vi "MSScript_Transform_Boolean.vi"(11 "Check_Str":string) -> (2 "Value Error?":bool, 3 "Value Output":bool)   [LabVIEW 2018, in "MSScript.lvclass"]
uses:
  MSScript.lvclass
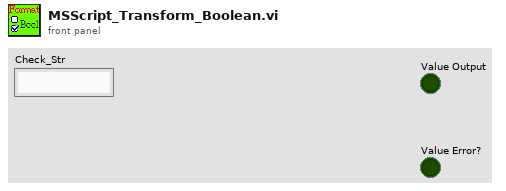
[diagram p1: front panel]
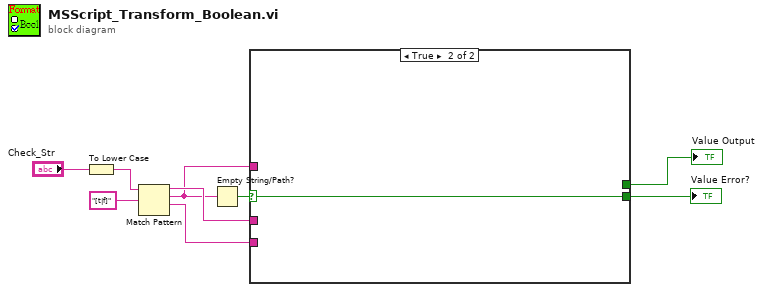
[diagram p0: block diagram]
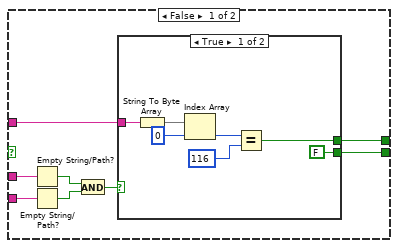
[diagram p2: hidden frame]
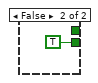
[diagram p3: hidden frame]
diagram:
  n1 = To Lower Case(string="Check_Str") -> (all lower case string=w1:string)
  n2 = Match Pattern(string=w1, regular expression="[t|f]") -> (before substring=w7:string, match substring=w5:string, after substring=w6:string)  [unwired: 1 in, 1 out]
  n3 = Empty String/Path?(string/path=w5) -> (empty?=w8:bool)
  n4 = case shown="True" w8 {
    selector: w8 -> [_ w26]
    tunnel: [w12 w26] -> w4
    tunnel: w7 -> [w14 _]
    tunnel: w6 -> [w15 _]
    tunnel: w5 -> [w11 _]
    tunnel: [w10 _] -> w3
    frame False {
      n5 = Empty String/Path?(string/path=w14) -> (empty?=w16:bool)
      n6 = Empty String/Path?(string/path=w15) -> (empty?=w17:bool)
      n7 = And(x=w16, y=w17) -> (x .and. y?=w13:bool)
      n8 = case shown="True" w13 {
        tunnel: [FALSE TRUE] -> w12
        tunnel: w11 -> [w24 _]
        tunnel: [w19 _] -> w10
        frame True {
          n9 = String To Byte Array(string=w24) -> (unsigned byte array=w23:u8[])
          n10 = Index Array(array=w23, index=0) -> (element=w21:u8)
          n11 = Equal?(x=w21, y=u8 116) -> (x = y?=w19:bool)
        }
        frame False {
        }
      }
    }
    frame True {
    }
  }
  "Value Error?" <- w4
  "Value Output" <- w3
